vi "Run.vi"   [LabVIEW 2010]
uses:
  BehaviorClassification.lvclass
  TrialBasedExperimentObject/TrialBasedExperiment.lvclass
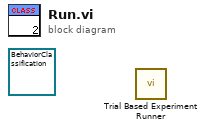
[diagram p0: block diagram]
diagram:
  (unwired) refnum<class "BehaviorClassification.lvclass"> refnum ("BehaviorClassification.lvclass")
  n1 = call "Trial Based Experiment Runner.vi"() -> ()  [unwired: 12 in]
